vi "point-by-point speed and angle.vi"(6 "encoder fixed offest":sgl, 7 "filter torque":bool, 8 "speed history in":u32[](array[numeric])=[0, 0, 0, 0, 0, 0, 0, 0, 0, 0, 0, 0, 0, 0, 0, 0, 0, 0, 0, 0, 0, 0, 0, 0, 0, 0, 0, 0, 0, 0, 0, 0, 0, 0, 0, 0, 0, 0, 0, 0], 10 "angle pulse":u32, 11 "speed pulse":u32) -> (0 "speed history out":u32[](array[numeric]), 2 "calculated angle (radians)":sgl, 3 "calculated speed (rad/tick)":sgl)   [LabVIEW 2018]
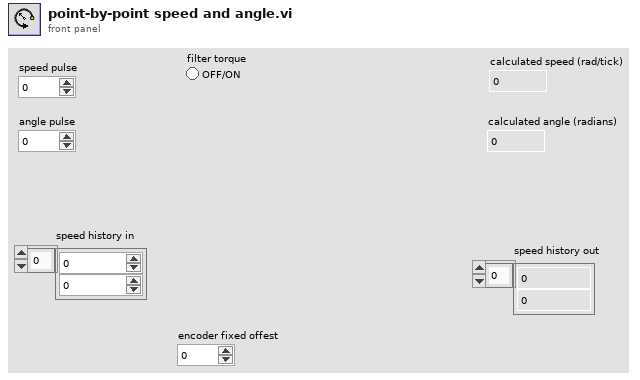
[diagram p1: front panel]
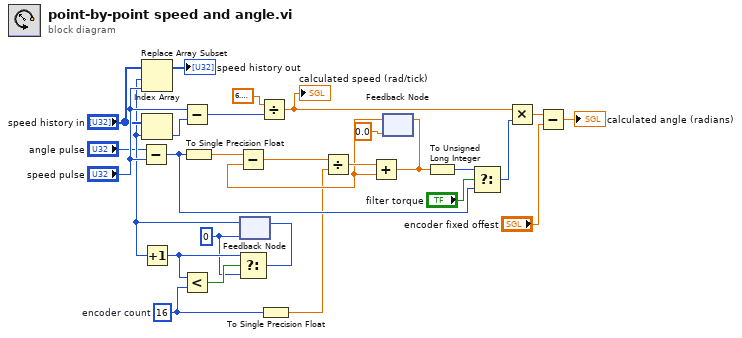
[diagram p0: block diagram]
diagram:
  w2 = i16 16  # encoder count
  w20 = i16 0
  n1 = Subtract(x="angle pulse", y="speed pulse") -> (x-y=w4:u32)
  n2 = To Single Precision Float(number=w4) -> (single precision float=w13:sgl)
  n3 = feedback #1(w20) -> (w23:i16)
  n4 = Replace Array Subset(array="speed history in", new element="speed pulse", index=w23) -> (→"speed history out":u32[])
  n5 = Index Array(array="speed history in", index=w23) -> (element=w27:u32)
  n6 = Increment(x=w23) -> (x+1=w21:i16)
  n7 = Subtract(x="speed pulse", y=w27) -> (x-y=w26:u32)
  n8 = Less?(x=w21, y=w2) -> (x < y?=w22:bool)
  n9 = Select(t=w21, s=w22, f=w20) -> (s? t:f=w19:i16)
  n10 = feedback-in #1(w19) -> ()
  n11 = Divide(x=sgl 6.2831855, y=w26) -> (x/y=w17:sgl)
  "calculated speed (rad/tick)" <- w17
  n12 = To Single Precision Float(number=w2) -> (single precision float=w1:sgl)
  n13 = feedback #2(sgl 0.0) -> (w9:sgl)
  n14 = Subtract(x=w13, y=w9) -> (x-y=w12:sgl)
  n15 = Divide(x=w12, y=w1) -> (x/y=w11:sgl)
  n16 = Add(x=w11, y=w9) -> (x+y=w8:sgl)
  n17 = feedback-in #2(w8) -> ()
  n18 = To Unsigned Long Integer(number=w8) -> (unsigned 32bit integer=w7:u32)
  n19 = Select(t=w7, s="filter torque", f=w4) -> (s? t:f=w3:u32)
  n20 = Multiply(x=w17, y=w3) -> (x*y=w16:sgl)
  n21 = Subtract(x=w16, y="encoder fixed offest") -> (x-y=→"calculated angle (radians)":sgl)
